vi "Fdx Create UDP Port (TX-SAP).vi"(6 "source info":T1, 8 "error in (no error)":errorcluster, 9 "VlId":u16, 10 "SapPort Config":T3={"partitionID"=0, "SubVlId"=0, "UdpSrcPort"=1, "UdpNumBufMessages"=0, "UdpMaxMessageSize"=1000}, 11 "port handle in":u32) -> (0 "error out":errorcluster, 1 "computedAddresses":T2 {"MACsrc" format="%.0x"}, 2 "sapPort handle out":u32, 3 "port handle out":u32)   [LabVIEW 2020, in "AIM664LV.lvlib"]
uses:
  AIM664LV.lvlib
  _controls/sap_config_tx.ctl
  _controls/comm_computedMAC-IP.ctl
  helpers/EthFrameManagement/controls/mac_src_info_afdx.ctl
  helpers/EthFrameManagement/controls/ip_src_info_afdx.ctl
  helpers/EthFrameManagement/EthFrameManagement.lvlib
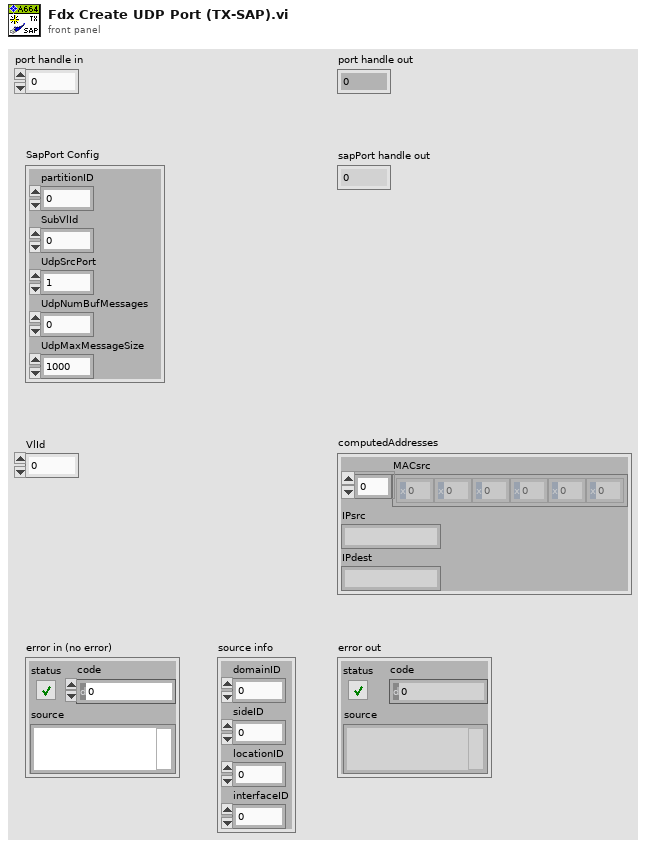
[diagram p1: front panel]
types:
  T1 = typedef "EthFrameManagement.lvlib/mac_src_info_afdx.ctl" = cluster{"domainID":u8, "sideID":u8, "locationID":u8, "interfaceID":u8}
  T2 = typedef "AIM664LV.lvlib/comm_computedMAC-IP.ctl" = cluster{"MACsrc":u8[], "IPsrc":string, "IPdest":string}
  T3 = typedef "AIM664LV.lvlib/sap_config_tx.ctl" = cluster{"partitionID":u8, "SubVlId":u8, "UdpSrcPort":u16, "UdpNumBufMessages":u32, "UdpMaxMessageSize":u32}
  T4 = cluster{"UdpSrc":u32, "IpSrc":u32, "VlId":u32, "SubVlId":u32, "UdpNumBufMessages":u32, "UdpMaxMessageSize":u32}
  T5 = typedef "EthFrameManagement.lvlib/ip_src_info_afdx.ctl" = cluster{"domainID":u8, "sideID":u8, "locationID":u8, "partitionID":u8}
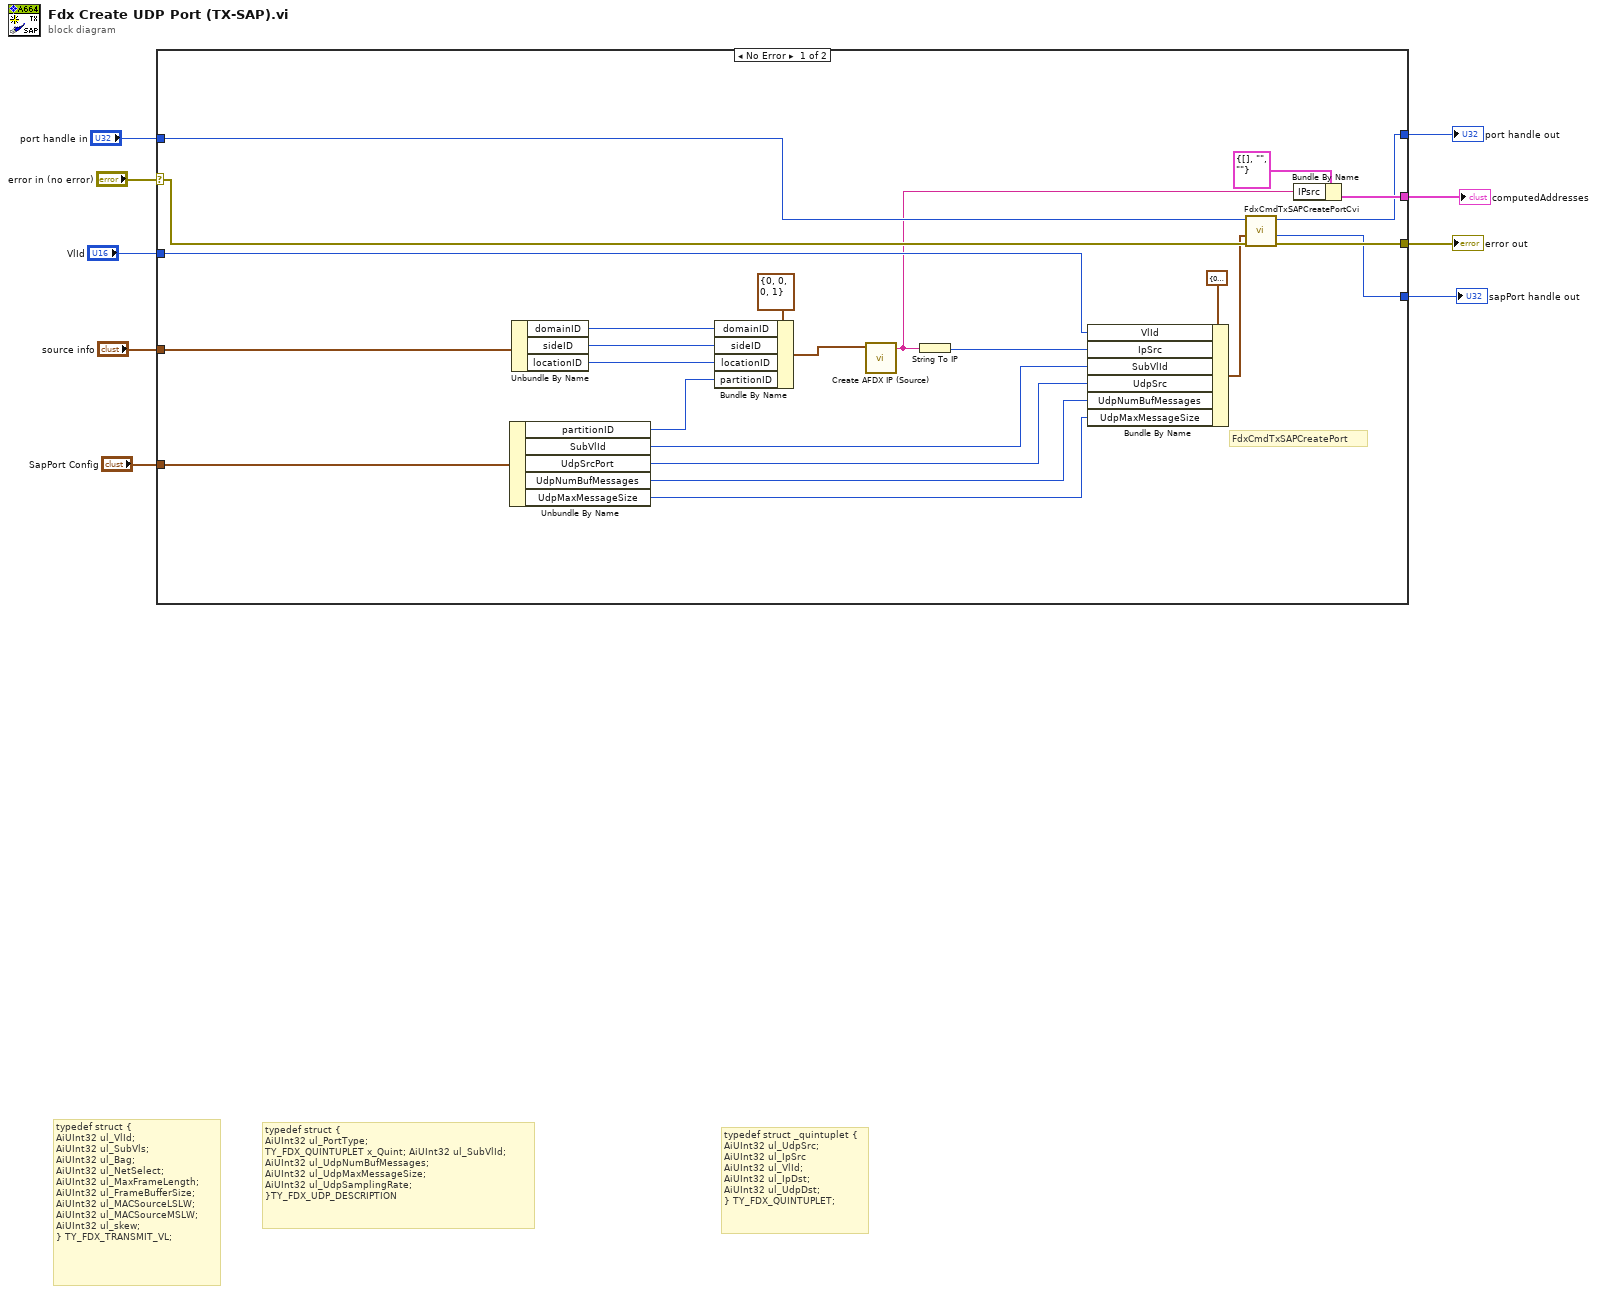
[diagram p0: block diagram]
diagram:
  # "typedef struct _quintuplet {\nAiUInt32 ul_UdpSrc;\nAiUInt32 ul_IpSrc\nAiUInt32 ul_VlId;\nAiUInt32 ul_IpDst;\nAiUInt32 ul_UdpDst;\n} TY_FDX_QUINTUPLET;"
  # "typedef struct {\nAiUInt32 ul_PortType;\nTY_FDX_QUINTUPLET x_Quint; AiUInt32 ul_SubVlId;\nAiUInt32 ul_UdpNumBufMessages;\nAiUInt32 ul_UdpMaxMessageSize;\nAiUInt32 ul_UdpSamplingRate;\n}TY_FDX_UDP_DESCRIPTION"
  # "typedef struct {\nAiUInt32 ul_VlId;\nAiUInt32 ul_SubVls;\nAiUInt32 ul_Bag;\nAiUInt32 ul_NetSelect;\nAiUInt32 ul_MaxFrameLength;\nAiUInt32 ul_FrameBufferSize;\nAiUInt32 ul_MACSourceLSLW;\nAiUInt32 ul_MACSourceMSLW;\nAiUInt32 ul_skew;\n} TY_FDX_TRANSMIT_VL;"
  n1 = case shown="No Error" "error in (no error)" {
    selector: "error in (no error)" -> [w32 w34]
    tunnel: "port handle in" -> [w33 w35]
    tunnel: [w12 w35] -> w7
    tunnel: [w28 w34] -> w6
    tunnel: "SapPort Config" -> [w31 _]
    tunnel: [w30 _] -> w4
    tunnel: [w11 _] -> w3
    tunnel: "VlId" -> [w29 _]
    tunnel: "source info" -> [w10 _]
    frame No Error {
      # "FdxCmdTxSAPCreatePort"
      n2 = Unbundle By Name(w31) -> ("partitionID"=w23:u8, "SubVlId"=w13:u8, "UdpSrcPort"=w15:u16, "UdpNumBufMessages"=w17:u32, "UdpMaxMessageSize"=w16:u32)
      n3 = Unbundle By Name(w10) -> ("domainID"=w22:u8, "sideID"=w21:u8, "locationID"=w20:u8)
      n4 = Bundle By Name(cluster=T5 {"domainID"=0, "sideID"=0, "locationID"=0, "partitionID"=1} ("Source Info"), "domainID"=w22, "sideID"=w21, "locationID"=w20, "partitionID"=w23) -> (w26:T5)
      n5 = call "Create AFDX IP (Source).vi"("Source Info"=w26) -> ("ip address"=w24:string)  [unwired: 10 in]
      n6 = String To IP(1:w24) -> (0:w14:u32)
      n7 = Bundle By Name(cluster=T4 {"UdpSrc"=0, "IpSrc"=0, "VlId"=0, "SubVlId"=0, "UdpNumBufMessages"=0, "UdpMaxMessageSize"=0} ("SapCreateIn"), "VlId"=w29, "IpSrc"=w14, "SubVlId"=w13, "UdpSrc"=w15, "UdpNumBufMessages"=w17, "UdpMaxMessageSize"=w16) -> (w19:T4)
      n8 = call "FdxCmdTxSAPCreatePortCvi.vi"("error in"=w32, "SapCreateIn"=w19, "InstrumentHandle"=w33) -> ("error out"=w28:errorcluster, "UdpHandle"=w11:u32, "InstrumentHandle"=w12:u32)  [unwired: 6 in]
      n9 = Bundle By Name(cluster=T2 {"MACsrc"=[], "IPsrc"="", "IPdest"=""} ("computedAddresses"), "IPsrc"=w24) -> (w30:T2)
    }
    frame Error {
    }
  }
  "port handle out" <- w7
  "sapPort handle out" <- w3
  "error out" <- w6
  "computedAddresses" <- w4
